vi "Get Direction.vi"(8 "error in (no error)":errorcluster, 10 "DUT1":bool, 11 "Measured signal":digitalwaveform(waveform)) -> (0 "error out":errorcluster, 2 "Stopped":bool, 3 "CW/CCW":bool)   [LabVIEW 2023]
uses:
  <vilib>/Waveform/DWDTOps.llb/DWDT Digital Signal Subset.vi
  <vilib>/Waveform/DWDTOps.llb/DWDT Search for Digital Pattern.vi
panel:
  out "A graph 2":digitalwaveform(graph)
  out "index A":dbl format="%0.2f"
  out "index B":dbl format="%0.2f"
  out "B graph":digitalwaveform(graph)
  out "A graph":digitalwaveform(graph)
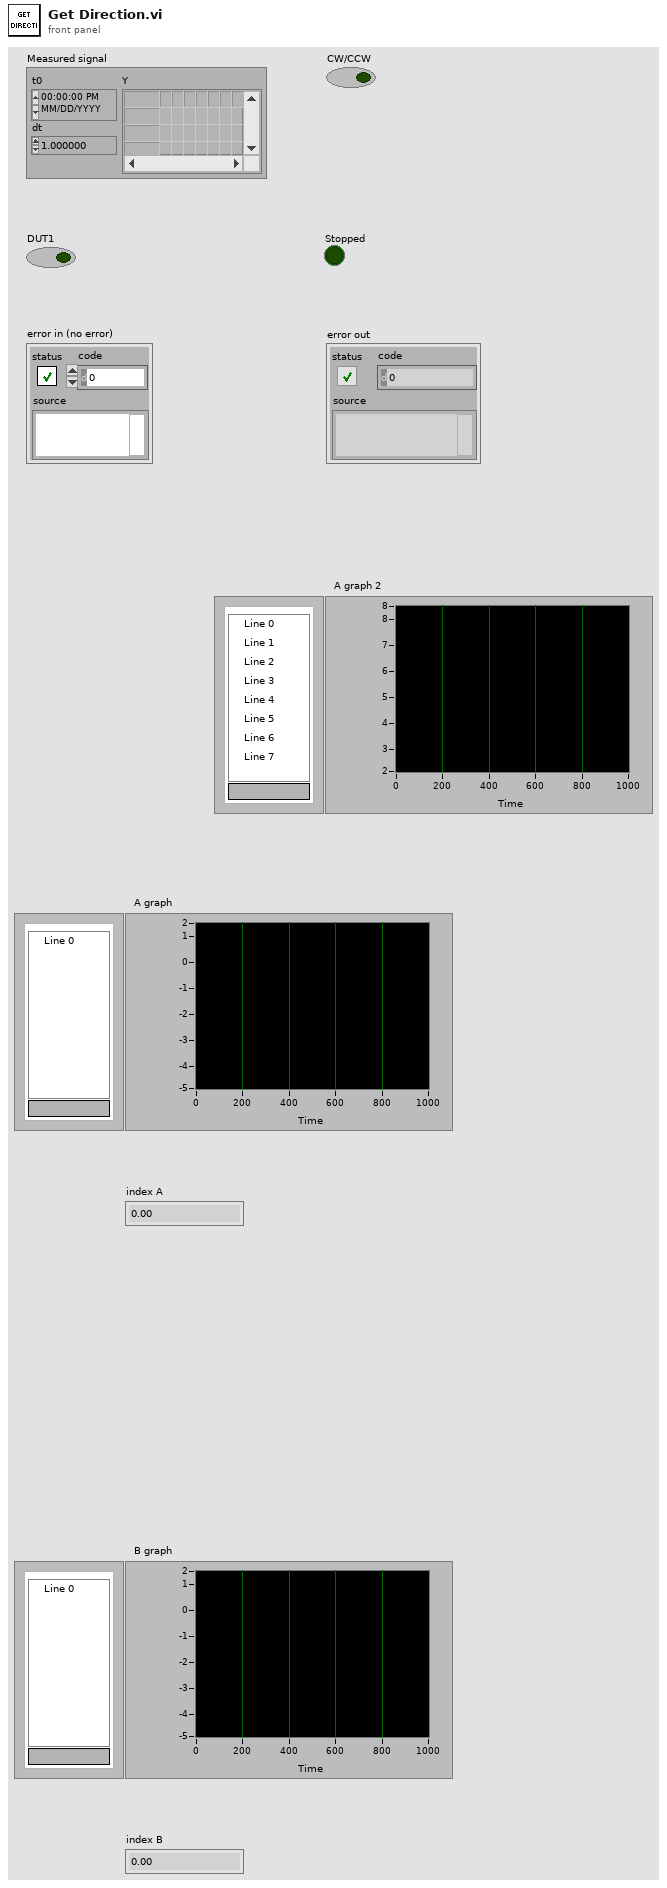
[diagram p1: front panel]
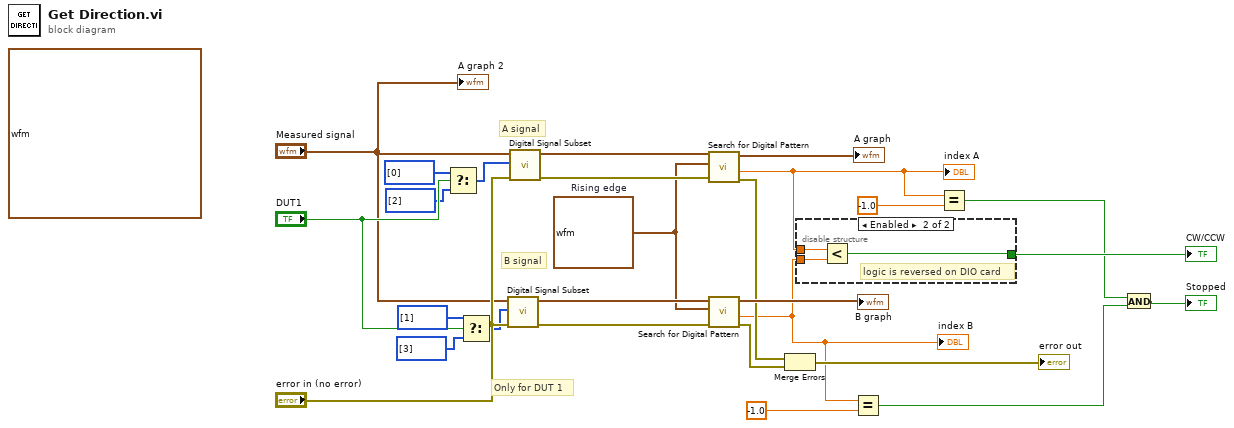
[diagram p0: block diagram]
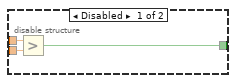
[diagram p2: hidden frame]
diagram:
  (unwired) digitalwaveform[] [{"t0"=timestamp(0 s since 1904-01-01), "dt"=0.0, "Y"={"transitions"=[], "data"=[[1, 0, 0, 0, 1, 0, 1, 0], [1, 0, 0, 0, 1, 0, 1, 0], [1, 0, 0, 0, 1, 0, 1, 0], [1, 0, 0, 0, 1, 0, 1, 0], [1, 0, 0, 0, 1, 0, 1, 0], [1, 0, 0, 0, 1, 0, 1, 0], [1, 0, 0, 0, 1, 0, 1, 0], [1, 0, 0, 0, 1, 0, 1, 0], [1, 0, 0, 0, 1, 0, 1, 0], [1, 0, 0, 0, 1, 0, 1, 0], [1, 0, 0, 0, 1, 0, 1, 0], [1, 0, 0, 0, 1, 0, 1, 0], [1, 0, 0, 0, 1, 0, 1, 0], [1, 0, 0, 0, 1, 0, 1, 0], [1, 0, 0, 0, 1, 0, 1, 0], [1, 0, 0, 0, 1, 0, 1, 0], [1, 0, 0, 0, 1, 0, 1, 0], [1, 0, 0, 0, 1, 0, 1, 0], [1, 0, 0, 0, 0, 0, 1, 0], [1, 0, 0, 0, 0, 0, 1, 0], [1, 0, 0, 0, 0, 0, 1, 0], [1, 0, 0, 0, 0, 0, 1, 0], [1, 0, 0, 0, 0, 0, 1, 0], [1, 0, 0, 0, 0, 0, 1, 0], [1, 0, 0, 0, 0, 0, 1, 0], [1, 0, 0, 0, 0, 0, 1, 0], [1, 0, 0, 0, 0, 0, 1, 0], [1, 0, 0, 0, 0, 0, 1, 0], [1, 0, 0, 0, 0, 0, 1, 0], [1, 0, 0, 0, 0, 0, 1, 0], [1, 0, 0, 0, 0, 0, 1, 0], [1, 0, 0, 0, 0, 0, 1, 0], [1, 0, 0, 0, 0, 0, 1, 0], [1, 0, 0, 0, 0, 0, 1, 0], [1, 0, 0, 0, 0, 0, 1, 0], [1, 0, 0, 0, 0, 0, 1, 0], [1, 0, 0, 0, 0, 0, 1, 0], [1, 0, 0, 0, 0, 0, 1, 0], [1, 0, 0, 0, 0, 0, 1, 0], [1, 0, 0, 0, 0, 0, 1, 0], [1, 0, 0, 0, 0, 0, 1, 0], [1, 0, 0, 0, 0, 0, 1, 0], [1, 0, 0, 0, 0, 0, 1, 0], [1, 0, 0, 0, 0, 1, 1, 0], [1, 0, 0, 0, 0, 1, 1, 0], [1, 0, 0, 0, 0, 1, 1, 0], [1, 0, 0, 0, 0, 1, 1, 0], [1, 0, 0, 0, 0, 1, 1, 0], [1, 0, 0, 0, 0, 1, 1, 0], [1, 0, 0, 0, 0, 1, 1, 0], [1, 0, 0, 0, 0, 1, 1, 0], [1, 0, 0, 0, 0, 1, 1, 0], [1, 0, 0, 0, 0, 1, 1, 0], [1, 0, 0, 0, 0, 1, 1, 0], [1, 0, 0, 0, 0, 1, 1, 0], [1, 0, 0, 0, 0, 1, 1, 0], [1, 0, 0, 0, 0, 1, 1, 0], [1, 0, 0, 0, 0, 1, 1, 0], [1, 0, 0, 0, 0, 1, 1, 0], [1, 0, 0, 0, 0, 1, 1, 0], [1, 0, 0, 0, 0, 1, 1, 0], [1, 0, 0, 0, 0, 1, 1, 0], [1, 0, 0, 0, 0, 1, 1, 0], [1, 0, 0, 0, 0, 1, 1, 0], [1, 0, 0, 0, 0, 1, 1, 0], [1, 0, 0, 0, 0, 1, 1, 0], [1, 0, 0, 0, 0, 1, 1, 0], [1, 0, 0, 0, 0, 1, 1, 0], [1, 0, 0, 0, 0, 1, 1, 0], [1, 0, 0, 0, 1, 1, 1, 0], [1, 0, 0, 0, 1, 1, 1, 0], [1, 0, 0, 0, 1, 1, 1, 0], [1, 0, 0, 0, 1, 1, 1, 0], [1, 0, 0, 0, 1, 1, 1, 0], [1, 0, 0, 0, 1, 1, 1, 0], [1, 0, 0, 0, 1, 1, 1, 0], [1, 0, 0, 0, 1, 1, 1, 0], [1, 0, 0, 0, 1, 1, 1, 0], [1, 0, 0, 0, 1, 1, 1, 0], [1, 0, 0, 0, 1, 1, 1, 0], [1, 0, 0, 0, 1, 1, 1, 0], [1, 0, 0, 0, 1, 1, 1, 0], [1, 0, 0, 0, 1, 1, 1, 0], [1, 0, 0, 0, 1, 1, 1, 0], [1, 0, 0, 0, 1, 1, 1, 0], [1, 0, 0, 0, 1, 1, 1, 0], [1, 0, 0, 0, 1, 0, 1, 0], [1, 0, 0, 0, 1, 0, 1, 0], [1, 0, 0, 0, 1, 0, 1, 0], [1, 0, 0, 0, 1, 0, 1, 0], [1, 0, 0, 0, 1, 0, 1, 0], [1, 0, 0, 0, 1, 0, 1, 0], [1, 0, 0, 0, 1, 0, 1, 0], [1, 0, 0, 0, 1, 0, 1, 0], [1, 0, 0, 0, 1, 0, 1, 0], [1, 0, 0, 0, 1, 0, 1, 0], [1, 0, 0, 0, 1, 0, 1, 0], [1, 0, 0, 0, 1, 0, 1, 0], [1, 0, 0, 0, 1, 0, 1, 0], [1, 0, 0, 0, 1, 0, 1, 0]]}}] ("Digital Waveform Graph")
  w16 = digitaldata {"transitions"=[], "data"=[[0], [1]]}  # Rising edge
  # "Only for DUT 1"
  # "B signal"
  # "A signal"
  n1 = Select(t=i32[] [0] ("signals"), s="DUT1", f=i32[] [2] ("signals")) -> (s? t:f=w14:i32[])
  n2 = Select(t=i32[] [1] ("signals"), s="DUT1", f=i32[] [3] ("signals")) -> (s? t:f=w13:i32[])
  n3 = call-poly <vilib>:"Digital Signal Subset.vi"("error in (no error)"="error in (no error)", "signals"=w13, "digital waveform"="Measured signal") -> ("error out"=w19:errorcluster, "digital subset"=w21:digitalwaveform)  [unwired: 7 in]
  n4 = call-poly <vilib>:"Digital Signal Subset.vi"("error in (no error)"="error in (no error)", "signals"=w14, "digital waveform"="Measured signal") -> ("error out"=w20:errorcluster, "digital subset"=w17:digitalwaveform)  [unwired: 7 in]
  n5 = call-poly <vilib>:"Search for Digital Pattern.vi"("error in (no error)"=w20, "digital pattern"=w16, "digital waveform in"=w17) -> ("error out"=w24:errorcluster, "index/time of pattern"=w5:dbl, "digital waveform out"=→"A graph":digitalwaveform)  [unwired: 6 in]
  "index A" <- w5
  n6 = call-poly <vilib>:"Search for Digital Pattern.vi"("error in (no error)"=w19, "digital pattern"=w16, "digital waveform in"=w21) -> ("error out"=w23:errorcluster, "index/time of pattern"=w8:dbl, "digital waveform out"=→"B graph":digitalwaveform)  [unwired: 6 in]
  "index B" <- w8
  n7 = Merge Errors(w24, w23) -> (→"error out":errorcluster)
  n8 = disable-structure shown="Enabled" {
    disable-tunnel: [w30 w31] -> w27
    disable-tunnel: w8 -> [w29 w32]
    disable-tunnel: w5 -> [w28 w33]
    frame Disabled {
      n9 = Greater?(x=w28, y=w29) -> (0:w30:bool)
    }
    frame Enabled {
      # "logic is reversed on DIO card"
      n10 = Less?(x=w33, y=w32) -> (x < y?=w31:bool)
    }
  }
  "CW/CCW" <- w27
  n11 = Equal?(x=w8, y=-1.0) -> (x = y?=w3:bool)
  n12 = Equal?(x=w5, y=-1.0) -> (x = y?=w4:bool)
  n13 = And(x=w4, y=w3) -> (x .and. y?=→"Stopped":bool)
  "A graph 2" <- "Measured signal"
